vi "LabVIEW Type to JSON Tree.vi"(8 "error in (no error)":errorcluster, 10 "Ctl Refnum":refnum<vi>) -> (0 "error out":errorcluster, 3 "JSON Tree Out":variant)   [LabVIEW 2013, in "i3-json.lvlib"]
uses:
  i3-json.lvlib
  JSON Types/JSON Type.ctl
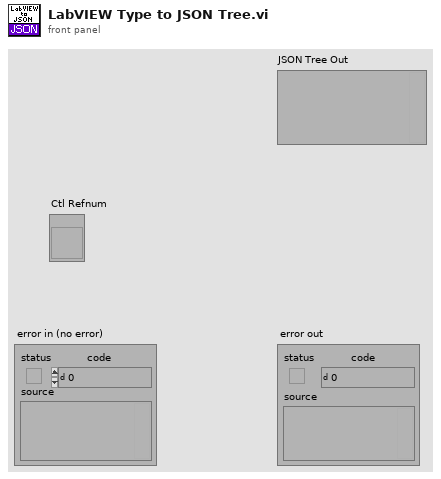
[diagram p1: front panel]
types:
  T1 = typedef "i3-json.lvlib/JSON Type.ctl" = enum8{"JSON Compatible", "JSON Array", "JSON Object", "JSON Null", "Double", "String", "Boolean", "Unknown", "Data JSON string"}
  T2 = typedef "Type Enum.ctl" = enum8{"Void", "I8", "I16", "I32", "I64", "U8", "U16", "U32", "U64", "Single Float", "Double Float", "Extended Float", "Single Complex", "Double Complex", "Extended Complex", "Enum I8 NEVER", "Enum I16 NEVER", "Enum I32 NEVER", "Enum I64 NEVER", "Enum U8", "Enum U16", "Enum U32", "Enum U64", "Single Float With Unit", "Double Float With Unit", "Extended Float With Unit", "Single Complex With Unit", "Double Complex With Unit", "Extended Complex With Unit", "boolU16", "Boolean", "String", "Handle", "Path", "Picture", "C String", "Pascal String", "Tag", "SubString", "Array", "SubArray", "Cluster", "Numeric Cluster", "Variant", "LV Variant", "Measure Data (waveform)", "Refnum", "ExtData", "function", "Typedef", "Poly VI", "bad wire", "LabVIEW Class Instance"}
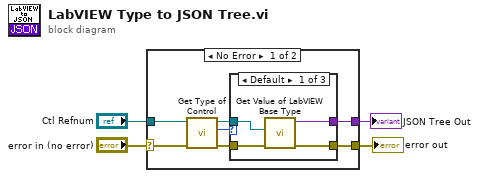
[diagram p0: block diagram]
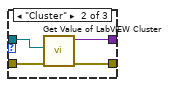
[diagram p2: hidden frame]
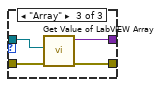
[diagram p3: hidden frame]
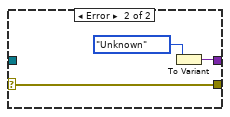
[diagram p4: hidden frame]
diagram:
  n1 = case shown="No Error" "error in (no error)" {
    selector: "error in (no error)" -> [w11 w26]
    tunnel: "Ctl Refnum" -> [w10 _]
    tunnel: [w6 w26] -> w2
    tunnel: [w5 w25] -> w1
    frame No Error {
      n2 = call <vilib>:"Get Type of Control.vi"("error in (no error)"=w11, "Control Ref In"=w10) -> ("error out"=w7:errorcluster, "Type Enum"=w9:T2, "Control Ref Out"=w8:refnum<vi>)  [unwired: 7 in]
      n3 = case shown="Default" w9 {
        tunnel: w8 -> [w13 w17 w21]
        tunnel: w7 -> [w15 w18 w22]
        tunnel: [w14 w19 w23] -> w6
        tunnel: [w12 w16 w20] -> w5
        frame Default {
          n4 = call "Get Value of LabVIEW Base Type.vi"("LabVIEW Base Type"=w13, "error in (no error)"=w15) -> ("JSON Tree Out"=w12:variant, "error out"=w14:errorcluster)  [unwired: 7 in]
        }
        frame "Cluster" {
          n5 = call "Get Value of LabVIEW Cluster.vi"("error in (no error)"=w18, "LabVIEW Cluster"=w17) -> ("error out"=w19:errorcluster, "JSON Tree Object Out"=w16:variant)  [unwired: 8 in]
        }
        frame "Array" {
          n6 = call "Get Value of LabVIEW Array.vi"("LabVIEW Array"=w21, "error in (no error)"=w22) -> ("JSON Tree Array"=w20:variant, "error out"=w23:errorcluster)  [unwired: 7 in]
        }
      }
    }
    frame Error {
      n7 = To Variant(anything=JSON_Type."Unknown" ("JSON Type")) -> (Variant=w25:variant)
    }
  }
  "error out" <- w2
  "JSON Tree Out" <- w1
